vi "Init from WebSocket.vi"(8 "error in (no error)":errorcluster) -> (0 "error out":errorcluster, 3 "FormulaG API out":refnum<class "FormulaG API.lvclass">)   [LabVIEW 2020]
uses:
  <vilib>/IlluminatedG/IG WebSocket Stream/Stream-Websocket/Websocket Server/Websocket Server.lvclass
  FormulaG API.lvclass
  <vilib>/IlluminatedG/IG WebSocket Stream/Stream-Websocket/Websocket Client/Websocket Client.lvclass
  <vilib>/IlluminatedG/lv-stream/stream/Stream.lvclass
  <vilib>/IlluminatedG/IG GodotServer/GodotLV/GodotServer/GodotServer.lvclass
panel:
  in  "Godot":refnum<class "GodotServer.lvclass">
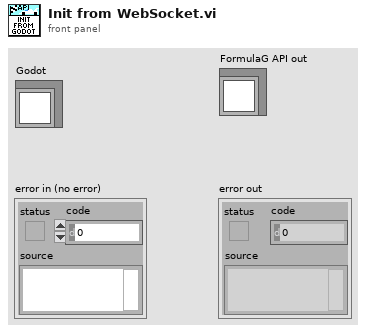
[diagram p1: front panel]
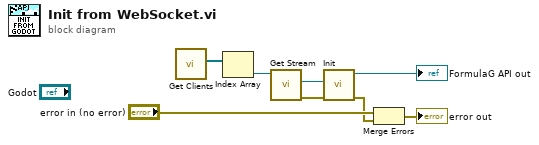
[diagram p0: block diagram]
diagram:
  n1 = call <vilib>:"Get Clients.vi"() -> ("Clients"=w6:refnum<class "Websocket Client.lvclass">[])  [unwired: 9 in, 2 out]
  n2 = Index Array(array=w6) -> (element=w5:refnum<class "Websocket Client.lvclass">)  [unwired: 1 in]
  n3 = call-dynamic "Get Stream.vi"("Websocket Client in"=w5) -> ("error out"=w3:errorcluster, "Stream"=w4:refnum<class "Stream.lvclass">)  [unwired: 8 in, 1 out]
  n4 = call "Init.vi"("error in (no error)"=w3, "Godot"=w4) -> ("error out"=w1:errorcluster, "FormulaG API out"=→"FormulaG API out":refnum<class "FormulaG API.lvclass">)  [unwired: 8 in]
  n5 = Merge Errors("error in (no error)", w1) -> (→"error out":errorcluster)
